vi "Pluvimätre.vi"(8 "Mise à zéro du niveau d'eau":bool=TRUE, 9 "data":bool caption="Indicateur lumineux") -> (2 "Quantité de pluie (en mm)":dbl)   [LabVIEW 2017]
uses:
  ae57919f-e50e-4202-b2a5-905aa4171cb0.vi
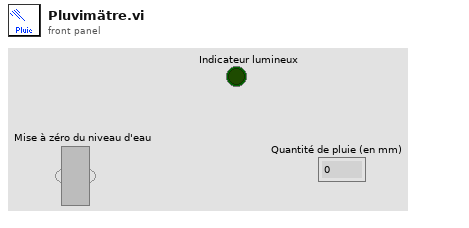
[diagram p1: front panel]
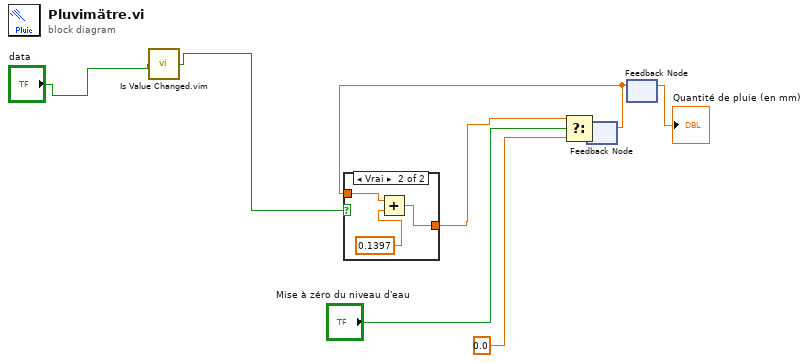
[diagram p0: block diagram]
diagram:
  n1 = call "Is Value Changed.vim"("value"="data") -> ("changed or first call?"=w6:bool)
  n2 = feedback #1() -> (w1:dbl)  [unwired: 1 in]
  n3 = case shown="Vrai" w6 {
    tunnel: w1 -> [w9 w10]
    tunnel: [w9 w12] -> w5
    frame False {
    }
    frame True {
      n4 = Add(x=w10, y=0.1397) -> (x+y=w12:dbl)
    }
  }
  n5 = Select(t=w5, s="Mise à zéro du niveau d'eau", f=0.0) -> (s? t:f=w3:dbl)
  n6 = feedback-in #1(w3) -> ()
  n7 = feedback #2() -> (→"Quantité de pluie (en mm)":dbl)  [unwired: 1 in]
  n8 = feedback-in #2(w1) -> ()
